vi "Read component configuration.vi"(8 "error in":errorcluster, 10 "initial configuration":refnum<class "TBM module configuration.lvclass">, 11 "Component in":refnum<class "Asynchronous Module Editor Node.lvclass">) -> (0 "error out":errorcluster, 2 "configuration out":refnum<class "TBM module configuration.lvclass">, 3 "Component out":refnum<class "Asynchronous Module Editor Node.lvclass">)   [LabVIEW 2013, in "PL Framework Configuration Tool.lvlib" / "Asynchronous Module Editor Node.lvclass"]
uses:
  Asynchronous Module Editor Node.lvclass
  <vilib>/NI/Tag Bus Module Framework/module configuration/TBM module configuration.lvclass
  asynchronous execution module/configuration/asynchronous execution module configuration.lvclass
  asynchronous execution module/configuration/asynchronous execution module configuration.lvclass/asynchronous execution module configuration.ctl
  Module editor node/module editor node.lvclass
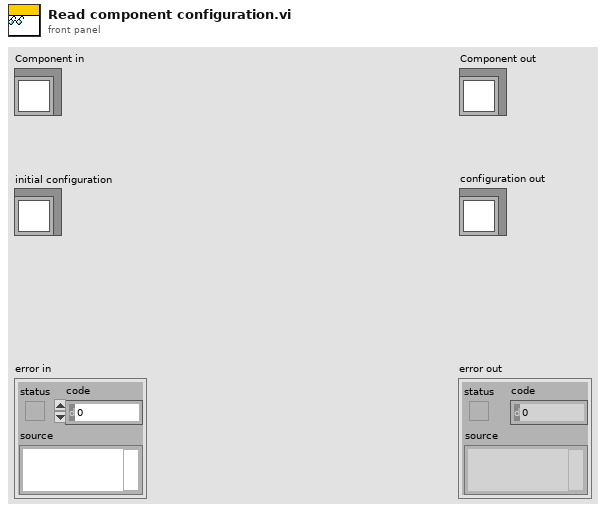
[diagram p1: front panel]
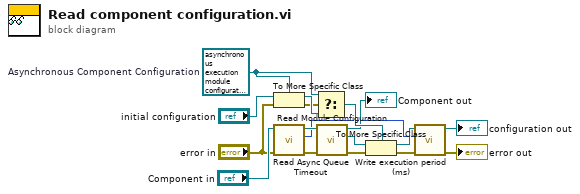
[diagram p0: block diagram]
diagram:
  w13 = refnum<class "asynchronous execution module configuration.lvclass"> refnum  # Asynchronous Component Configuration
  n1 = To More Specific Class(target class=w13, reference="initial configuration", error in="error in") -> (specific class reference=w15:refnum<class "asynchronous execution module configuration.lvclass">, error out=w14:errorcluster)
  n2 = call-dynamic "Read Async Queue Timeout.vi"("error in"="error in", "Module Editor Node in"="Component in") -> ("error out"=w7:errorcluster, "Queue Timeout"=w1:i32, "Module Editor Node out"=w12:refnum<class "Asynchronous Module Editor Node.lvclass">)  [unwired: 7 in]
  n3 = Select(t=w13, s=w14, f=w15) -> (s? t:f=w11:refnum<class "asynchronous execution module configuration.lvclass">)
  n4 = call "Read Module Configuration.vi"("error in"=w7, "Module Editor Node in"=w12) -> ("error out"=w4:errorcluster, "module configuration"=w10:refnum<class "TBM module configuration.lvclass">, "Module Editor Node out"=→"Component out":refnum<class "Asynchronous Module Editor Node.lvclass">)  [unwired: 7 in]
  n5 = To More Specific Class(target class=w11, reference=w10, error in=w4) -> (specific class reference=w6:refnum<class "asynchronous execution module configuration.lvclass">, error out=w5:errorcluster)
  n6 = call "Write execution period (ms).vi"("error in"=w5, "execution period (ms)"=w1, "Asynchronous Component Configuration in"=w6) -> ("error out"=→"error out":errorcluster, "Asynchronous Component Configuration out"=→"configuration out":refnum<class "asynchronous execution module configuration.lvclass">)  [unwired: 7 in]
